vi "Axes_N_Buttons.vi"() -> ()   [LabVIEW 2020]
panel:
  out "DrStart":bool
  out "DrBack":bool
  out "OpStart":bool
  out "OpBack":bool
  out "OpLeft":bool
  out "OpRight":bool
  out "OpDown":bool
  out "OpUp":bool
  out "AutoWheel":dbl
  out "AutoThrottle":dbl
  out "OpAxis5":dbl
  out "OpAxis4":dbl
  out "OpButtonRB":bool
  out "OpButtonLB":bool
  out "OpButtonY":bool
  out "OpButtonX":bool
  out "OpButtonB":bool
  out "OpButtonA":bool
  out "OpAxis3":dbl
  out "OpAxis2":dbl
  out "OpAxis1":dbl
  out "OpAxis0":dbl
  out "DrButtonRB":bool
  out "DrButtonLB":bool
  out "DrButtonY":bool
  out "DrButtonX":bool
  out "DrButtonB":bool
  out "DrButtonA":bool
  out "DrAxis4":dbl
  out "DrAxis3":dbl
  out "DrAxis2":dbl
  out "DrAxis1":dbl
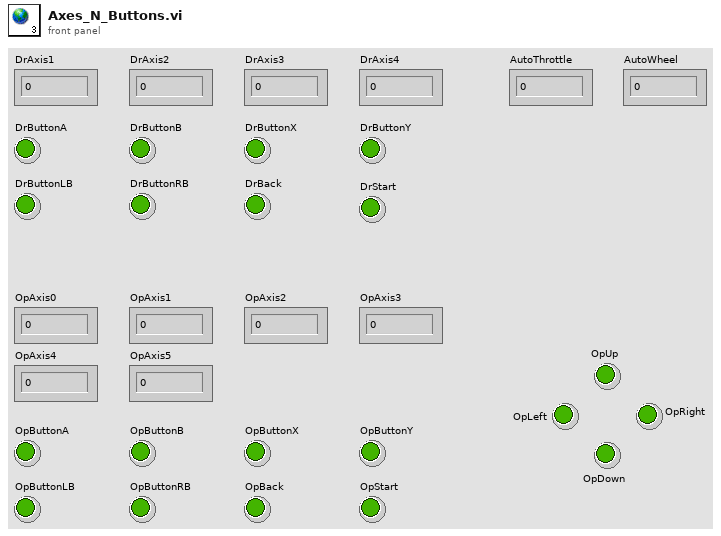
[diagram p1: front panel]
diagram:
